vi "read_data (SubVI).vi"(11 "data tasks":T2) -> (0 "sample rate":dbl, 1 "Rescaled data":i16[][](array[numeric]), 2 "Output data":dbl[][](array[numeric]), 3 "output data tasks":T1)   [LabVIEW 2014]
uses:
  <vilib>/DAQmx/read.llb/DAQmx Read (Analog 2D DBL NChan NSamp).vi
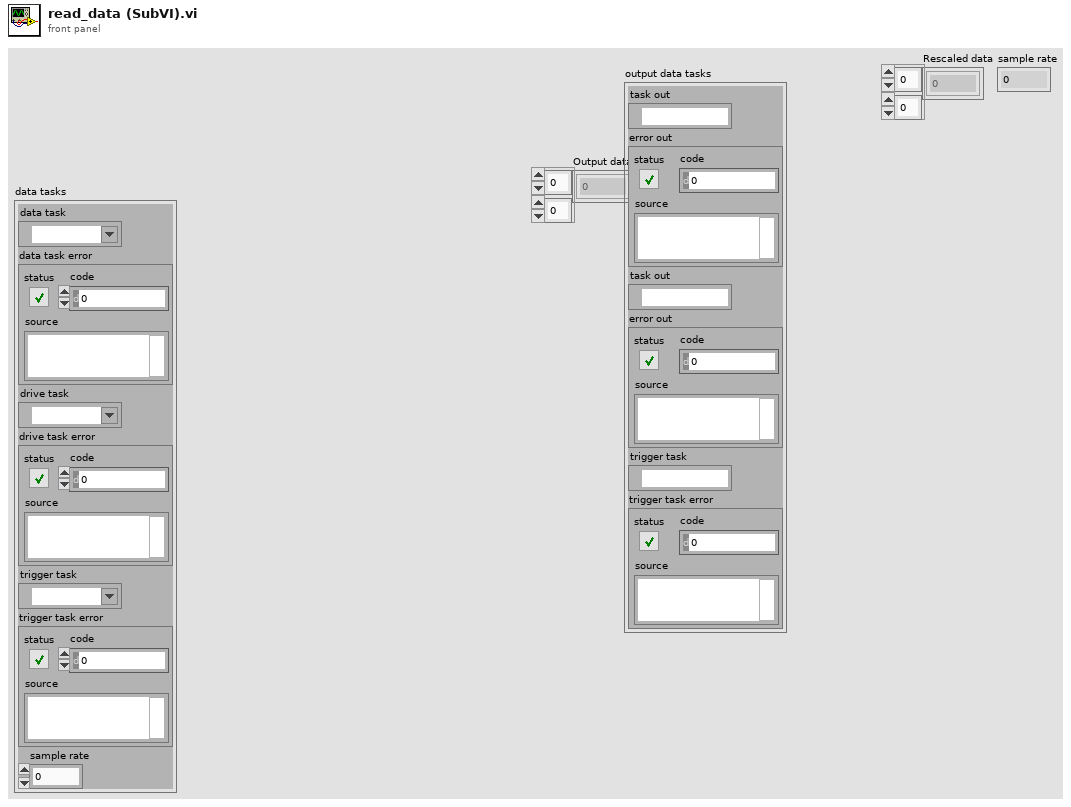
[diagram p1: front panel]
types:
  T1 = cluster{"task out":refnum<k21>, "error out":errorcluster, "task out":refnum<k21>, "error out":errorcluster, "trigger task":refnum<k21>, "trigger task error":errorcluster}
  T2 = cluster{"data task":refnum<k21>, "data task error":errorcluster, "drive task":refnum<k21>, "drive task error":errorcluster, "trigger task":refnum<k21>, "trigger task error":errorcluster, "sample rate":dbl}
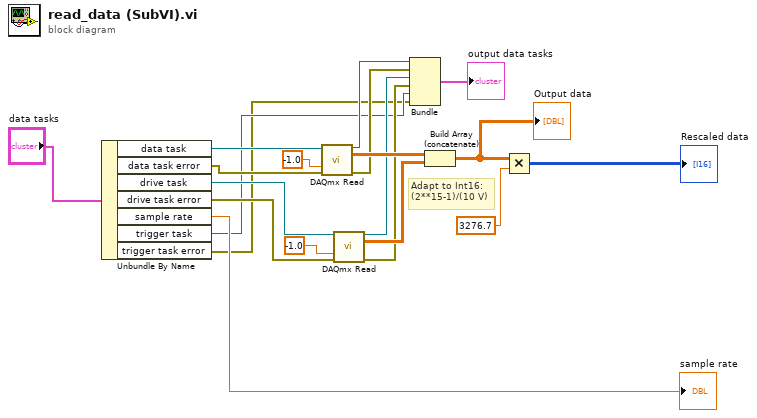
[diagram p0: block diagram]
diagram:
  # "Adapt to Int16: \n(2**15-1)/(10 V)"
  n1 = Unbundle By Name("data tasks") -> ("data task"=w19:refnum<k21>, "data task error"=w18:errorcluster, "drive task"=w16:refnum<k21>, "drive task error"=w15:errorcluster, "sample rate"=→"sample rate":dbl, "trigger task"=w4:refnum<k21>, "trigger task error"=w3:errorcluster)
  n2 = call-poly <vilib>:"DAQmx Read.vi"("task/channels in"=w19, "timeout"=-1.0, "error in"=w18) -> ("task out"=w8:refnum<k21>, "data"=w13:dbl[][], "error out"=w7:errorcluster)  [unwired: 10 in]
  n3 = call-poly <vilib>:"DAQmx Read.vi"("task/channels in"=w16, "timeout"=-1.0, "error in"=w15) -> ("task out"=w6:refnum<k21>, "data"=w12:dbl[][], "error out"=w5:errorcluster)  [unwired: 10 in]
  n4 = Bundle("task out"=w8, "error out"=w7, "task out"=w6, "error out"=w5, "trigger task"=w4, "trigger task error"=w3) -> (→"output data tasks":T1)  [unwired: 1 in]
  n5 = Build Array (concatenate)(w13, w12) -> (w9:dbl[][])
  "Output data" <- w9
  n6 = Multiply(x=w9, y=3276.7) -> (x*y=→"Rescaled data":i16[][])
